vi "Write background.vi"(8 "error in (no error)":errorcluster, 10 "background":dbl[](array[numeric]), 11 "Glaz-I in":refnum<class "Glaz.lvclass">) -> (0 "error out":errorcluster, 3 "Glaz-I out":refnum<class "Glaz.lvclass">)   [LabVIEW 2019, in "Glaz.lvclass"]
uses:
  Glaz.lvclass
  _cameraBase/_cameraBase.lvclass
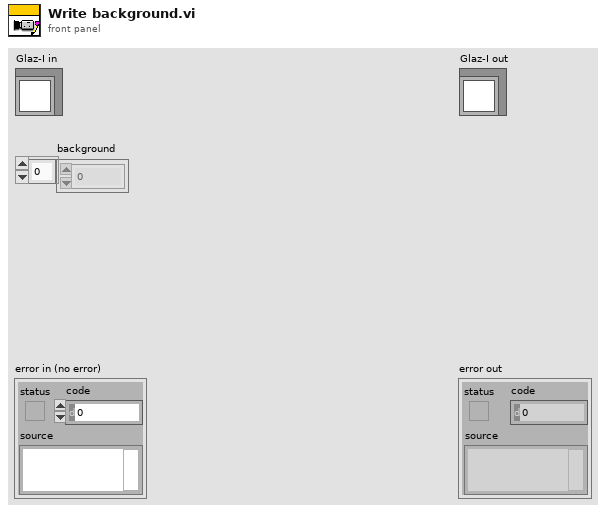
[diagram p1: front panel]
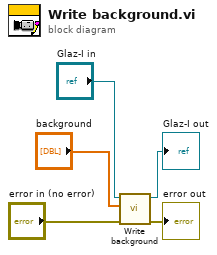
[diagram p0: block diagram]
diagram:
  n1 = call-parent "Write background.vi"("error in (no error)"="error in (no error)", "background"="background", "_cameraBase in"="Glaz-I in") -> ("error out"=→"error out":errorcluster, "_cameraBase out"=→"Glaz-I out":refnum<class "Glaz.lvclass">)  [unwired: 7 in]
